vi "Config_INTAN.vi"(0 "TCP Network Connection in":refnum<k5>, 1 "data in 2":string, 2 "data in 3":string, 3 "data in 4":string, 14 "error in (no error)":errorcluster, 19 "data in":string) -> (4 "data out":string, 5 "error out":errorcluster, 15 "data out 2":string, 16 "data out 3":string, 17 "data out 4":string)   [LabVIEW 2019]
panel:
  out "TCP Network Connection out":refnum<k5>
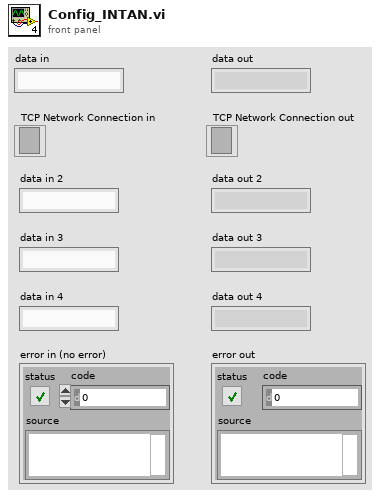
[diagram p1: front panel]
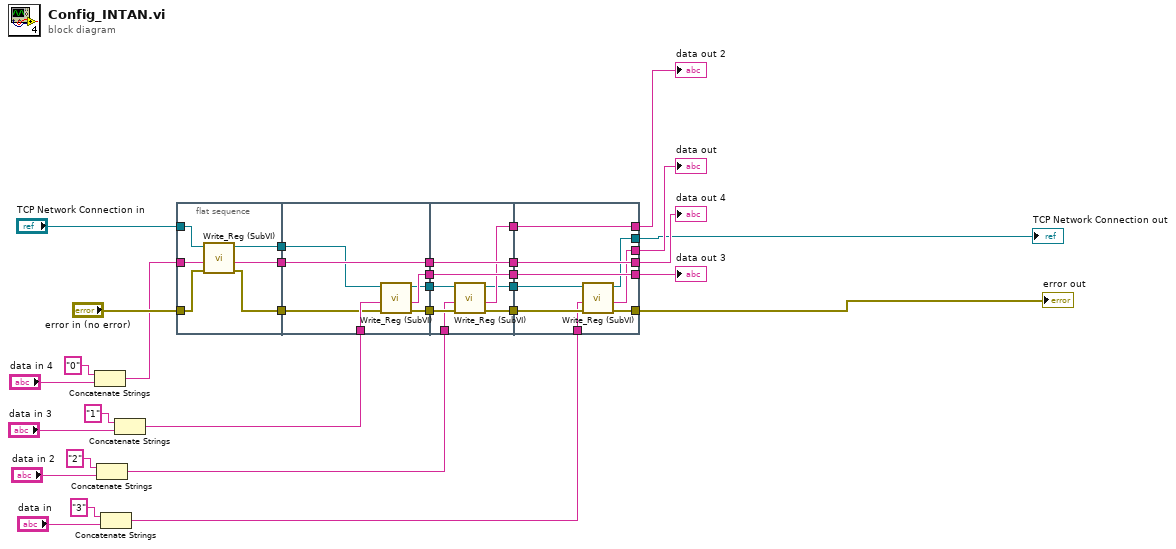
[diagram p0: block diagram]
diagram:
  n1 = Concatenate Strings("0" ("string"), "data in 4") -> (w23:string)
  n2 = Concatenate Strings("2" ("string"), "data in 2") -> (w3:string)
  n3 = Concatenate Strings("3" ("string"), "data in") -> (w7:string)
  n4 = Concatenate Strings("1" ("string"), "data in 3") -> (w19:string)
  n5 = flat-sequence {
    tunnel: "error in (no error)" -> [w38]
    tunnel: w23 -> [w37]
    tunnel: "TCP Network Connection in" -> [w36]
    tunnel: [w35] -> w20
    tunnel: [w34] -> w2
    tunnel: [w33] -> w1
    tunnel: w20 -> [w45]
    tunnel: w19 -> [w44]
    tunnel: [w45] -> w17
    tunnel: [w43] -> w16
    tunnel: [w42] -> w15
    tunnel: [w41] -> w14
    tunnel: w2 -> [w40]
    tunnel: w1 -> [w39]
    tunnel: w17 -> [w53]
    tunnel: w16 -> [w51]
    tunnel: w15 -> [w52]
    tunnel: w14 -> [w50]
    tunnel: [w53] -> w12
    tunnel: [w52] -> w11
    tunnel: [w49] -> w10
    tunnel: [w48] -> w9
    tunnel: [w47] -> w8
    tunnel: w3 -> [w46]
    tunnel: [w60] -> w13
    tunnel: [w61] -> w18
    tunnel: [w62] -> w21
    tunnel: w12 -> [w62]
    tunnel: w11 -> [w61]
    tunnel: w10 -> [w59]
    tunnel: w9 -> [w60]
    tunnel: w8 -> [w57]
    tunnel: w7 -> [w58]
    tunnel: [w56] -> w6
    tunnel: [w55] -> w5
    tunnel: [w54] -> w4
    frame #0 {
      n6 = call "Write_Reg (SubVI).vi"("error in (no error)"=w38, "data in"=w37, "TCP Network Connection in"=w36) -> ("error out"=w34:errorcluster, "data out"=w35:string, "TCP Network Connection out"=w33:refnum<k5>)  [unwired: 6 in]
    }
    frame #1 {
      n7 = call "Write_Reg (SubVI).vi"("error in (no error)"=w40, "data in"=w44, "TCP Network Connection in"=w39) -> ("error out"=w43:errorcluster, "data out"=w42:string, "TCP Network Connection out"=w41:refnum<k5>)  [unwired: 6 in]
    }
    frame #2 {
      n8 = call "Write_Reg (SubVI).vi"("error in (no error)"=w51, "data in"=w46, "TCP Network Connection in"=w50) -> ("error out"=w49:errorcluster, "data out"=w48:string, "TCP Network Connection out"=w47:refnum<k5>)  [unwired: 6 in]
    }
    frame #3 {
      n9 = call "Write_Reg (SubVI).vi"("error in (no error)"=w59, "data in"=w58, "TCP Network Connection in"=w57) -> ("error out"=w56:errorcluster, "data out"=w55:string, "TCP Network Connection out"=w54:refnum<k5>)  [unwired: 6 in]
    }
  }
  "data out" <- w5
  "data out 2" <- w13
  "data out 3" <- w18
  "TCP Network Connection out" <- w4
  "error out" <- w6
  "data out 4" <- w21
